vi "get channel names.vi"(0 "reference in":refnum<class "TDMS_DataHandler.lvclass">, 5 "error in (no error)":errorcluster) -> (14 "reference out":refnum<class "TDMS_DataHandler.lvclass">, 15 "Group name":string, 17 "channel names (out)":string[](array[string]), 19 "error out":errorcluster)   [LabVIEW 2019, in "TDMS_DataHandler.lvclass"]
doc: "Gets the channel name based on the provided groupname"
uses:
  TDMS_DataHandler.lvclass
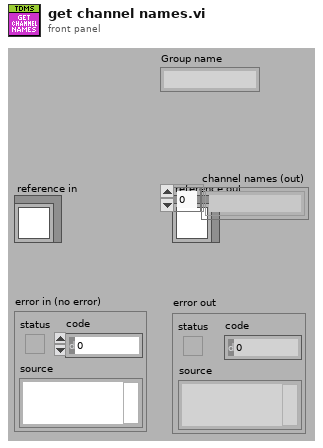
[diagram p1: front panel]
types:
  T1 = typedef "TDMS_DataHandler.lvclass/ObjectAttributesRef.ctl" = refnum<data-value>
  T2 = typedef "TDMS_DataHandler.lvclass/ObjectAttributes.ctl" = cluster{"Directory":path, "FilePath":path, "FileRef":refnum<k34>, "ExperimentName":string, "GroupName":string, "ChannelNames":string[], "Datum":waveform(dbl)[], "Group_Metadata":cluster{"property names":string[], "property values":variant[]}, "Channel_Metadata":cluster{"property names":string[], "property values":variant[]}}
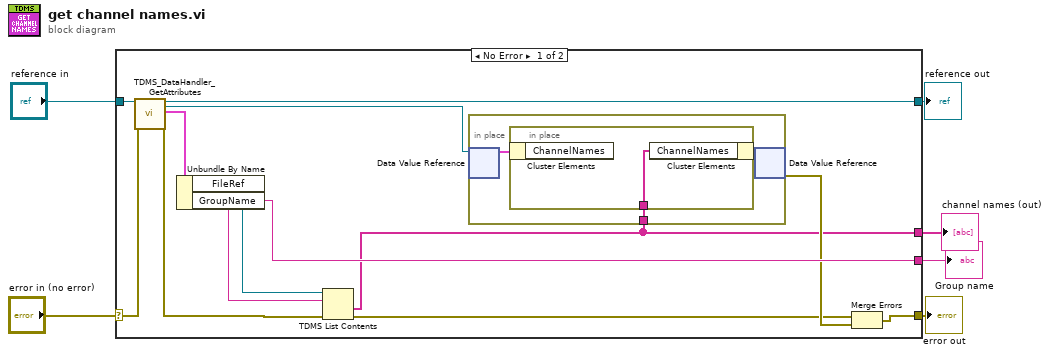
[diagram p0: block diagram]
diagram:
  n1 = case shown="No Error" "error in (no error)" {
    selector: "error in (no error)" -> [w18 w24]
    tunnel: [w9 w24] -> w5
    tunnel: [w17 w23] -> w3
    tunnel: "reference in" -> [w15 w23]
    tunnel: [w7 _] -> w2
    tunnel: [w12 _] -> w1
    frame No Error {
      n2 = call "TDMS_DataHandler_GetAttributes.vi"("reference in"=w15, "error in (no error)"=w18) -> ("reference out"=w17:refnum<class "TDMS_DataHandler.lvclass">, "attributes ref"=w8:T1, "attributes"=w16:T2, "error out"=w13:errorcluster)  [unwired: 14 in]
      n3 = Unbundle By Name(w16) -> ("FileRef"=w14:refnum<k34>, "GroupName"=w12:string)
      n4 = TDMS List Contents(4:w13, 6:w12, 7:w14) -> (0:w10:errorcluster, 1:w7:string[])  [unwired: 2 out]
      n5 = in-place {
        in-place-border: w7 -> [w19]
        n6 = in-place-dvr #1(w8) -> (w20:T2)  [unwired: 1 out]
        n7 = in-place {
          in-place-border: w19 -> [w22]
          n8 = in-place-cluster #2(w20) -> ()  [unwired: 1 out]
          n9 = in-place-cluster #2("ChannelNames"=w22) -> (w21:T2)
        }
        n10 = in-place-dvr #1(w21) -> (w11:errorcluster)  [unwired: 1 out]
      }
      n11 = Merge Errors(w10, w11) -> (w9:errorcluster)
    }
    frame Error {
    }
  }
  "error out" <- w5
  "reference out" <- w3
  "channel names (out)" <- w2
  "Group name" <- w1
